vi "aft_xmpl_Learning_Curve (MSE).vi"(1 "e(n)":dbl[][](array[numeric])) -> (0 "MSE":dbl[](array[numeric]))   [LabVIEW 2019]
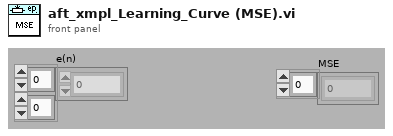
[diagram p1: front panel]
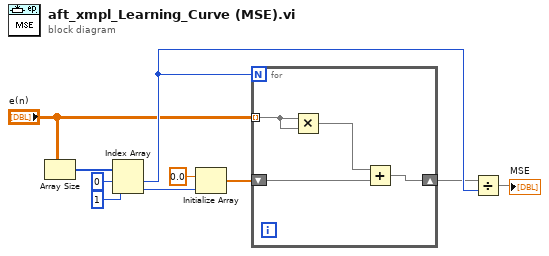
[diagram p0: block diagram]
diagram:
  n1 = Array Size(array="e(n)") -> (size(s)=w2:i32[])
  n2 = Index Array(array=w2, index #1=0 ("index"), index #2=1 ("index")) -> (element #1=w9:i32, element #2=w5:i32)
  n3 = Initialize Array(0.0 ("element"), w5) -> (w7:dbl[])
  n4 = for {
    N: w9 -> [_]
    tunnel: "e(n)" -> [w12] mode=indexing
    shift-right: [w13] -> w8
    shift-left: w7 -> [w14]
    n5 = Multiply(x=w12, y=w12) -> (x*y=w11:dbl[])
    n6 = Add(x=w11, y=w14) -> (x+y=w13:dbl[])
  }
  n7 = Divide(x=w8, y=w9) -> (x/y=→"MSE":dbl[])
